vi "X.vi"(11 "DataIn":T5) -> (3 "DataOut":T1)   [LabVIEW 2017]
doc: "SubVI criada para mostrar popup para o usuário indicando que o player X foi o vencedor."
uses:
  controls/DataIn.ctl
  controls/Tabuleiro.ctl
  controls/GameOption.ctl
  controls/Table.ctl
  controls/DataOut.ctl
panel:
  in  "Sair":bool
  in  "Jogar novamente":bool
  # "X é o vencedor!"
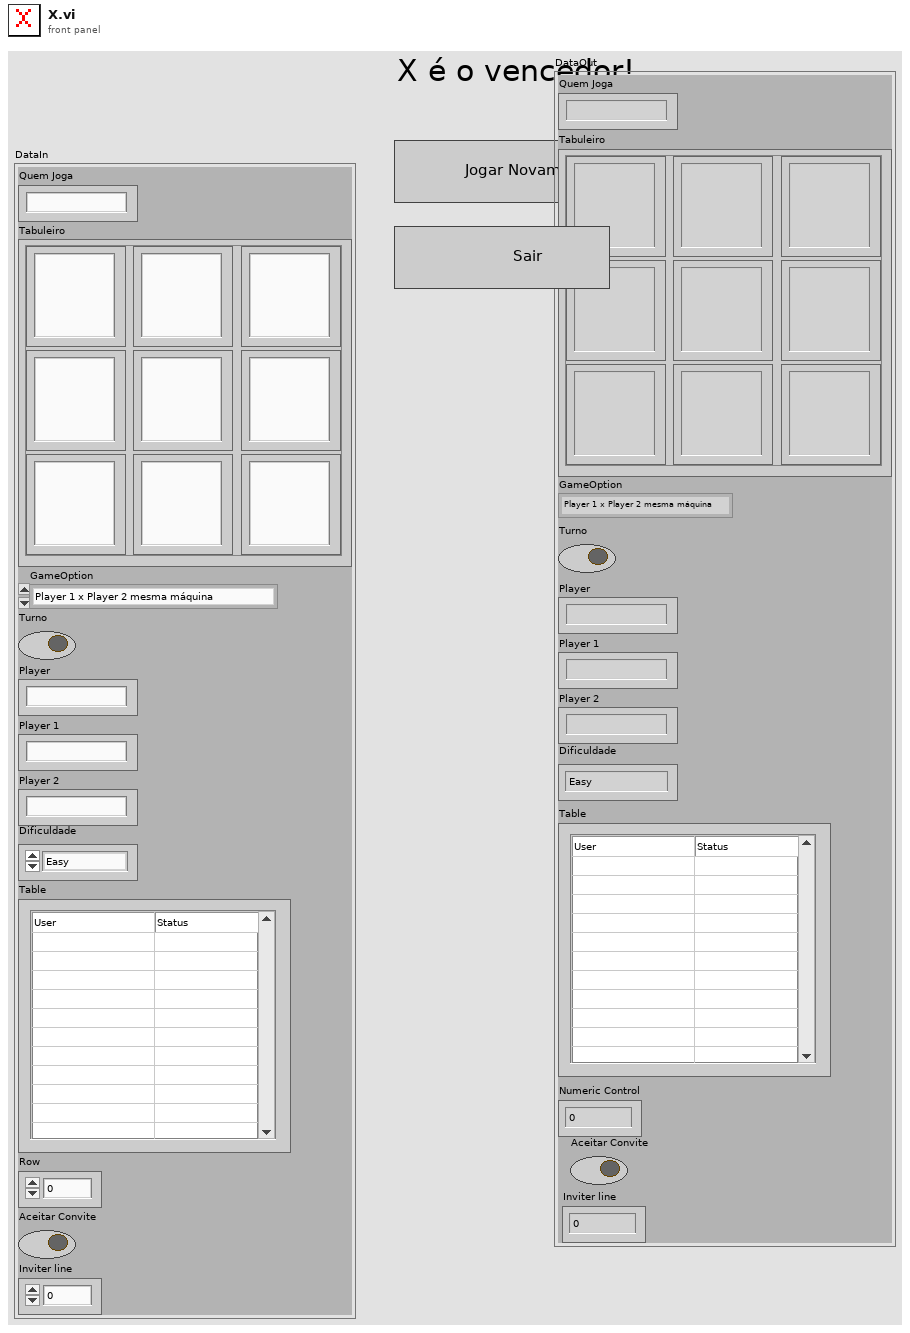
[diagram p1: front panel]
types:
  T1 = typedef "DataOut.ctl" = cluster{"Quem Joga":string, "Tabuleiro":T2, "GameOption":T3, "Turno":bool, "Player":string, "Player 1":string, "Player 2":string, "Dificuldade":enum16{"Easy", "Medium", "Hard"}, "Table":T4, "Numeric Control":u32, "Aceitar Convite":bool, "Inviter line":u32}
  T2 = typedef "Tabuleiro.ctl" = cluster{"(0,0)":string, "(1,0)":string, "(0,1)":string, "(1,1)":string, "(2,0)":string, "(1,2)":string, "(2,2)":string, "(0,2)":string, "(2,1) ":string}
  T3 = typedef "GameOption.ctl" = enum16{"Player 1 x Player 2 mesma máquina", "Player 1 x Player 2 pela rede", "Player 1 x Computador", "Wait for Event", "Initialize", "Stop"}
  T4 = typedef "Table.ctl" = string[][]
  T5 = typedef "DataIn.ctl" = cluster{"Quem Joga":string, "Tabuleiro":T2, "GameOption":T3, "Turno":bool, "Player":string, "Player 1":string, "Player 2":string, "Dificuldade":enum16{"Easy", "Medium", "Hard"}, "Table":T4, "Row":u32, "Aceitar Convite":bool, "Inviter line":u32}
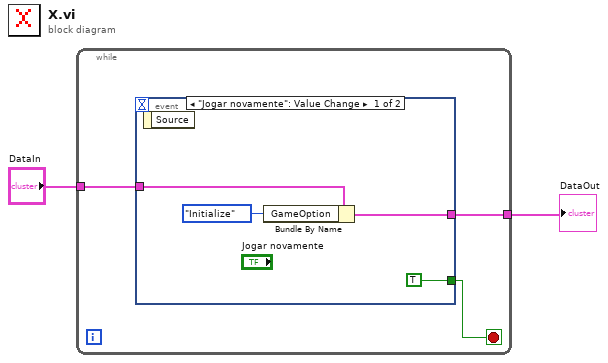
[diagram p0: block diagram]
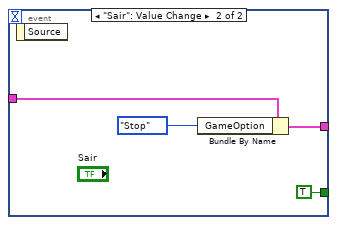
[diagram p2: hidden frame]
diagram:
  n1 = while {
    tunnel: "DataIn" -> [w4]
    tunnel: [w5] -> w1
    stop <- w3 stop-if-true
    n2 = event shown="[0] \"Jogar novamente\": Value Change" {
      selector: _ -> [_ _]
      dyn-events: _ -> [_ _]
      timeout: _ -> [_ _]
      tunnel: [w7 w13] -> w5
      tunnel: w4 -> [w8 w12]
      tunnel: [TRUE TRUE] -> w3
      event "Jogar novamente": Value Change {
        n3 = event-data() -> ()  [unwired: 1 in, 1 out]
        n4 = Bundle By Name(cluster=w8, "GameOption"=GameOption."Initialize") -> (w7:T5)
      }
      event "Sair": Value Change {
        n5 = event-data() -> ()  [unwired: 1 in, 1 out]
        n6 = Bundle By Name(cluster=w12, "GameOption"=GameOption."Stop") -> (w13:T5)
      }
    }
  }
  "DataOut" <- w1
